vi "2angleServo-WorkOnXYGraph.vi"() -> ()   [LabVIEW 2019]
uses:
  <vilib>/LabVIEW Interface for Arduino/Type Defs/Board Type.ctl
  <vilib>/LabVIEW Interface for Arduino/LabVIEW Interface for Arduino.lvlib
panel:
  out "vert":u8
  out "hor":u8
  out "XY Graph":cluster{"X":dbl, "Y":dbl}[](graph)
  out "err arduino":errorcluster
  in  "stop":bool
  in  "VISA resource":refnum<visa-resource-name>
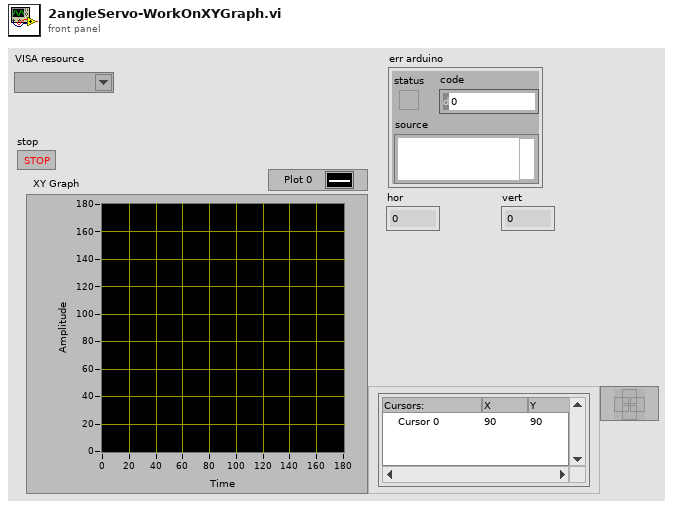
[diagram p1: front panel]
types:
  T1 = typedef "LabVIEW Interface for Arduino.lvlib/Board Type.ctl" = enum16{"Uno", "Dimuelanove w/Atmega 328", "Mega 2560"}
  T2 = typedef "LabVIEW Interface for Arduino.lvlib/Arduino Resource.ctl" = cluster{"VISA resource":refnum<visa-resource-name>, "Board Type":T1, "Connection Type":enum8{"USB / Serial"}, "Bytes Per Packet (15)":u8}
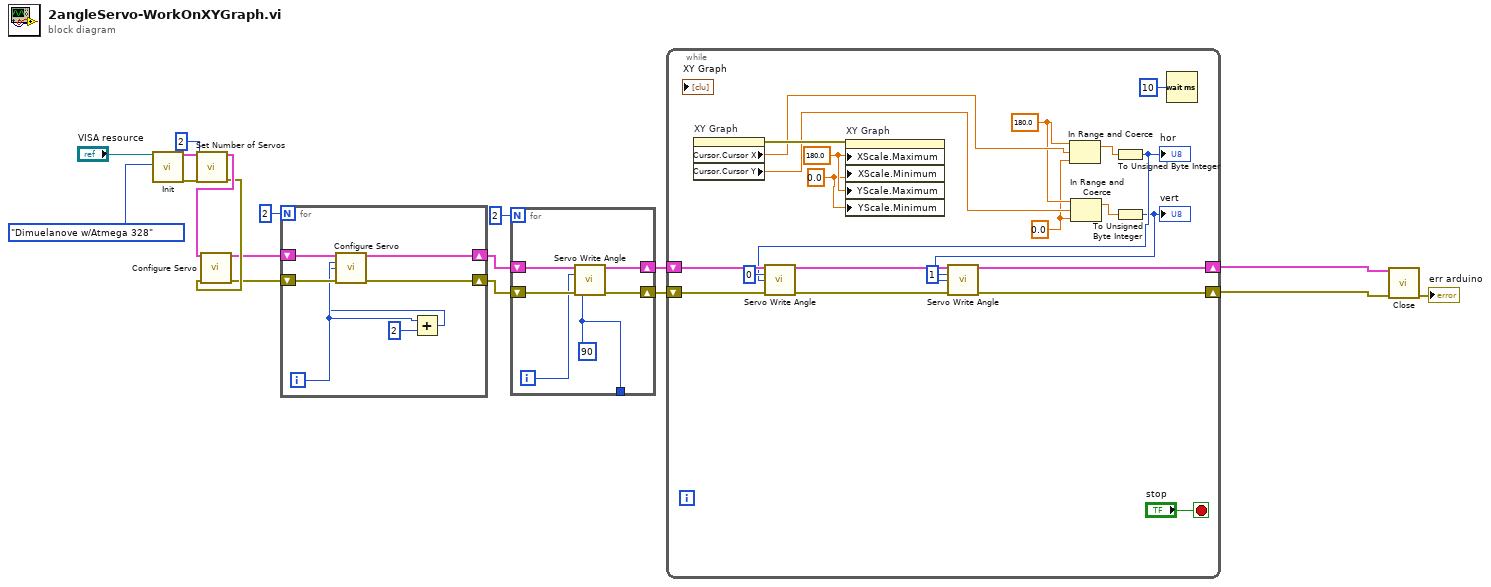
[diagram p0: block diagram]
diagram:
  n1 = call <vilib>:"Init.vi"("VISA resource"="VISA resource", "Board Type (Uno)"=Board_Type."Dimuelanove w/Atmega 328") -> ("Arduino Resource"=w16:T2, "error out"=w15:errorcluster)  [unwired: 16 in]
  n2 = call <vilib>:"Set Number of Servos.vi"("Arduino Resource"=w16, "Number Of Servos (1)"=u8 2, "error in"=w15) -> ("Arduino Resource"=w13:T2, "error out"=w12:errorcluster)  [unwired: 11 in]
  n3 = call <vilib>:"Configure Servo.vi"("Arduino Resource"=w13, "error in"=w12) -> ("Arduino Resource"=w11:T2, "error out"=w10:errorcluster)  [unwired: 12 in]
  n4 = for {
    N: 2 -> [_]
    shift-right: [w20] -> w8
    shift-left: w11 -> [w25]
    shift-right: [w19] -> w7
    shift-left: w10 -> [w24]
    i -> [w23]
    n5 = Add(x=w23, y=2) -> (x+y=w21:i32)
    n6 = call <vilib>:"Configure Servo.vi"("Arduino Resource"=w25, "Servo Number (0)"=w23, "DIO Pin (2)"=w21, "error in"=w24) -> ("Arduino Resource"=w20:T2, "error out"=w19:errorcluster)  [unwired: 10 in]
  }
  n7 = for {
    N: 2 -> [_]
    shift-right: [w29] -> w6
    shift-left: w8 -> [w31]
    shift-right: [w28] -> w5
    shift-left: w7 -> [w30]
    tunnel: [w26] -> _
    i -> [w27]
    w26 = u8 90 ("Angle (Degrees)")
    n8 = call <vilib>:"Servo Write Angle.vi"("Arduino Resource"=w31, "Servo Number"=w27, "Angle (Degrees)"=w26, "error in"=w30) -> ("Arduino Resource"=w29:T2, "error out"=w28:errorcluster)  [unwired: 10 in]
  }
  n9 = while {
    shift-right: [w39] -> w3
    shift-left: w6 -> [w41]
    shift-right: [w36] -> w2
    shift-left: w5 -> [w38]
    stop <- "stop" stop-if-true
    w44 = 0.0 ("lower limit")
    w45 = 180.0 ("upper limit")
    w49 = 0.0 ("X Scale.Range:Minimum")
    w50 = 180.0 ("X Scale.Range:Maximum")
    n10 = property on="XY Graph" class="XYGraph (strict)"() -> (error out=w48:errorcluster, "Cursor.Cursor X"=w47:dbl, "Cursor.Cursor Y"=w46:dbl)  [unwired: 2 in, 1 out]
    n11 = property on="XY Graph" class="XYGraph (strict)"(error in=w48, "XScale.Maximum"=w50, "XScale.Minimum"=w49, "YScale.Maximum"=w50, "YScale.Minimum"=w49) -> ()  [unwired: 1 in, 2 out]
    n12 = In Range and Coerce(upper limit=w45, x=w47, lower limit=w44) -> (coerced(x)=w42:dbl)  [unwired: 1 out]
    n13 = In Range and Coerce(upper limit=w45, x=w46, lower limit=w44) -> (coerced(x)=w43:dbl)  [unwired: 1 out]
    n14 = To Unsigned Byte Integer(number=w42) -> (unsigned 8bit integer=w34:u8)
    "hor" <- w34
    n15 = call <vilib>:"Servo Write Angle.vi"("Arduino Resource"=w41, "Servo Number"=u8 0, "Angle (Degrees)"=w34, "error in"=w38) -> ("Arduino Resource"=w40:T2, "error out"=w37:errorcluster)  [unwired: 10 in]
    n16 = To Unsigned Byte Integer(number=w43) -> (unsigned 8bit integer=w33:u8)
    "vert" <- w33
    n17 = call <vilib>:"Servo Write Angle.vi"("Arduino Resource"=w40, "Servo Number"=u8 1, "Angle (Degrees)"=w33, "error in"=w37) -> ("Arduino Resource"=w39:T2, "error out"=w36:errorcluster)  [unwired: 10 in]
    n18 = Wait (ms)(milliseconds to wait=u32 10) -> ()  [unwired: 1 out]
  }
  n19 = call <vilib>:"Close.vi"("Arduino Resource"=w3, "error in"=w2) -> ("error out"=→"err arduino":errorcluster)  [unwired: 13 in]
